vi "GetPathByPrototypeName.vi"(11 "prototype":string) -> (3 "path":path)   [LabVIEW 2017]
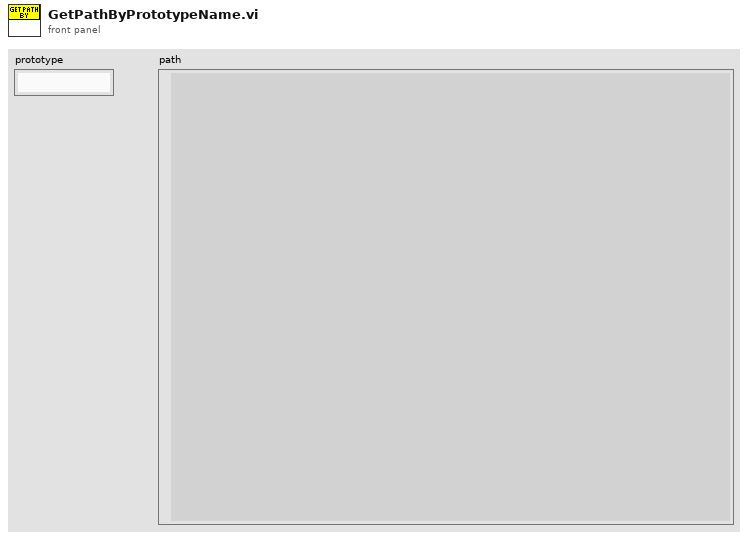
[diagram p1: front panel]
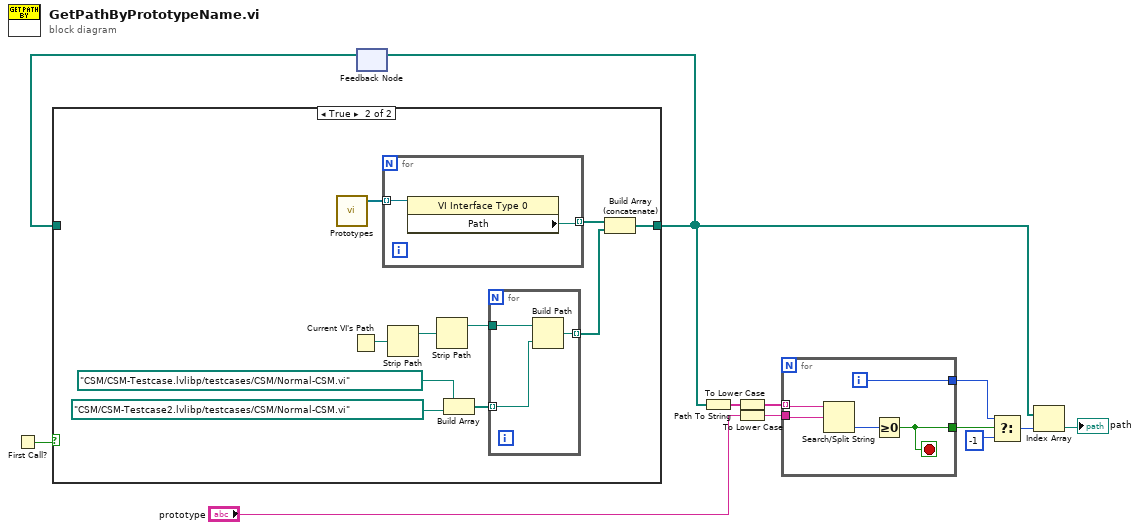
[diagram p0: block diagram]
diagram:
  n1 = First Call?() -> (First Call?: T/F=w3:bool)
  n2 = feedback #1() -> (w1:path[])  [unwired: 1 in]
  n3 = case shown="True" w3 {
    tunnel: [w13 w14] -> w2
    tunnel: w1 -> [w13 _]
    frame False {
    }
    frame True {
      n4 = call "Prototypes.vi"() -> ("prototypes"=w17:refnum<vi>[])  [unwired: 11 in]
      n5 = Current VI's Path() -> (path=w20:path)
      n6 = for {
        tunnel: w17 -> [w25] mode=indexing
        tunnel: [w24] -> w16 mode=indexing
        n7 = property class="VI Interface Type 0"(reference=w25) -> ("Path"=w24:path)  [unwired: 1 in, 2 out]
      }
      n8 = Strip Path(path=w20) -> (stripped path=w19:path)  [unwired: 1 out]
      n9 = Strip Path(path=w19) -> (stripped path=w18:path)  [unwired: 1 out]
      n10 = Build Array(path "CSM/CSM-Testcase.lvlibp/testcases/CSM/Normal-CSM.vi" ("vi path"), path "CSM/CSM-Testcase2.lvlibp/testcases/CSM/Normal-CSM.vi" ("vi path")) -> (w23:path[])
      n11 = for {
        tunnel: w18 -> [w27]
        tunnel: w23 -> [w28] mode=indexing
        tunnel: [w26] -> w15 mode=indexing
        n12 = Build Path(base path=w27, name or relative path=w28) -> (appended path=w26:path)
      }
      n13 = Build Array (concatenate)(w16, w15) -> (w14:path[])
    }
  }
  n14 = feedback-in #1(w2) -> ()
  n15 = Path To String(path=w2) -> (string=w12:string[])
  n16 = To Lower Case(string=w12) -> (all lower case string=w6:string[])
  n17 = To Lower Case(string="prototype") -> (all lower case string=w11:string)
  n18 = for {
    tunnel: w6 -> [w30] mode=indexing
    tunnel: w11 -> [w29]
    tunnel: [w33] -> w9
    tunnel: [w31] -> w10
    i -> [w33]
    stop <- w31 stop-if-true
    n19 = Search/Split String(string=w30, search string/char (-)=w29) -> (offset of match=w32:i32)  [unwired: 1 in, 2 out]
    n20 = Greater Or Equal To 0?(x=w32) -> (x >= 0?=w31:bool)
  }
  n21 = Select(t=w9, s=w10, f=-1) -> (s? t:f=w7:i32)
  n22 = Index Array(array=w2, index=w7) -> (element=→"path":path)
